vi "etc_XCITE_CloseDevice.vi"(2 "error in (no error)":errorcluster {"code" format="%x"}, 3 "h":u64) -> (0 "error out":errorcluster {"code" format="%x"})   [LabVIEW 2019, in "XCite.lvlib"]
doc: "Closes communication with the slelected X-cite device."
uses:
  XCite.lvlib
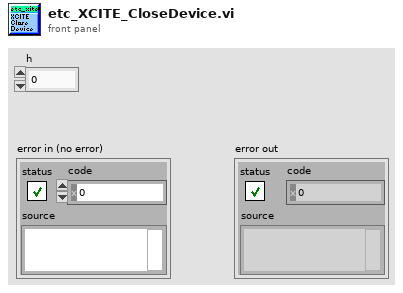
[diagram p1: front panel]
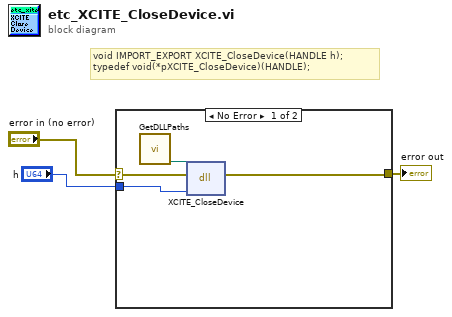
[diagram p0: block diagram]
diagram:
  # "void IMPORT_EXPORT XCITE_CloseDevice(HANDLE h);\ntypedef void(*pXCITE_CloseDevice)(HANDLE);"
  n1 = case shown="No Error" "error in (no error)" {
    selector: "error in (no error)" -> [w7 w8]
    tunnel: [w4 w8] -> w3
    tunnel: "h" -> [w6 _]
    frame No Error {
      n2 = call "GetDLLPaths.vi"() -> ("etc_xcite_path"=w5:path)  [unwired: 8 in, 3 out]
      n3 = dll-call lib="C:/LabVIEWDevFall2024/pco.labview/labview_sdk/runtime/bin64/etc_xcite.dll" fn="XCITE_CloseDevice"(path in=w5, error in=w7, "h"=w6) -> (error out=w4:errorcluster)  [unwired: 3 in, 1 out]
    }
    frame Error {
    }
  }
  "error out" <- w3
